vi "Baseline calculation_new.vi"(4 "Sampling rate":dbl=10000.0 format="%#_13g", 5 "Data type":T2 items=["AXON", "HEKA"], 7 "Event Detection (1D)":T1[](array[typedef])) -> (3 "Baseline info":cluster{dbl[][]}[](array[cluster]))   [LabVIEW 2017]
uses:
  Data type_new.ctl
  Event Detection cluster.ctl
  <vilib>/Analysis/baseanly.llb/Mean (DBL).vi
  <vilib>/Analysis/NI_AALBase.lvlib
  <vilib>/Analysis/NI_AALPro.lvlib
panel:
  out "Event Detection (1D) OUT":T1[](array[typedef])
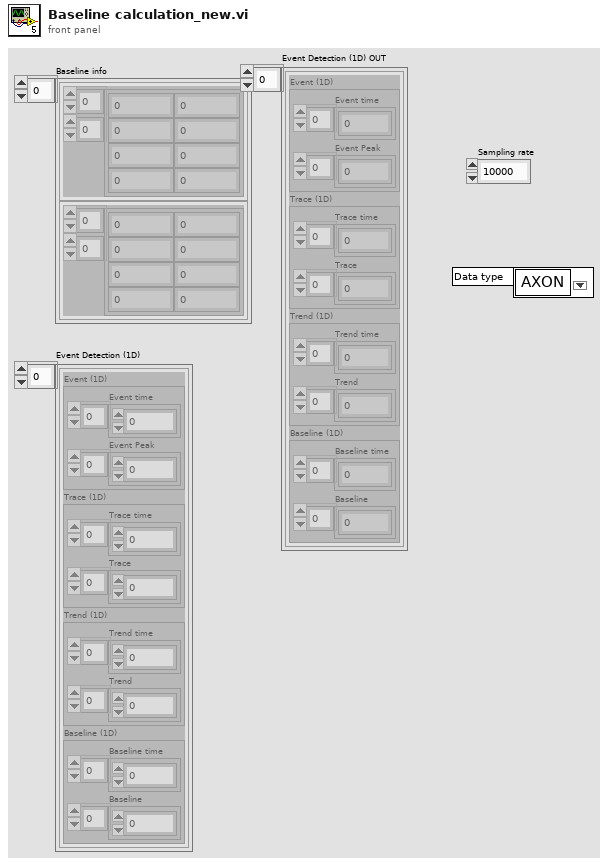
[diagram p1: front panel]
types:
  T1 = typedef "Event Detection cluster.ctl" = cluster{"Event (1D)":cluster{"Event time":dbl[], "Event Peak":dbl[]}, "Trace (1D)":cluster{"Trace time":dbl[], "Trace":dbl[]}, "Trend (1D)":cluster{"Trend time":dbl[], "Trend":dbl[]}, "Baseline (1D)":cluster{"Baseline time":dbl[], "Baseline":dbl[]}}
  T2 = typedef "Data type_new.ctl" = u16
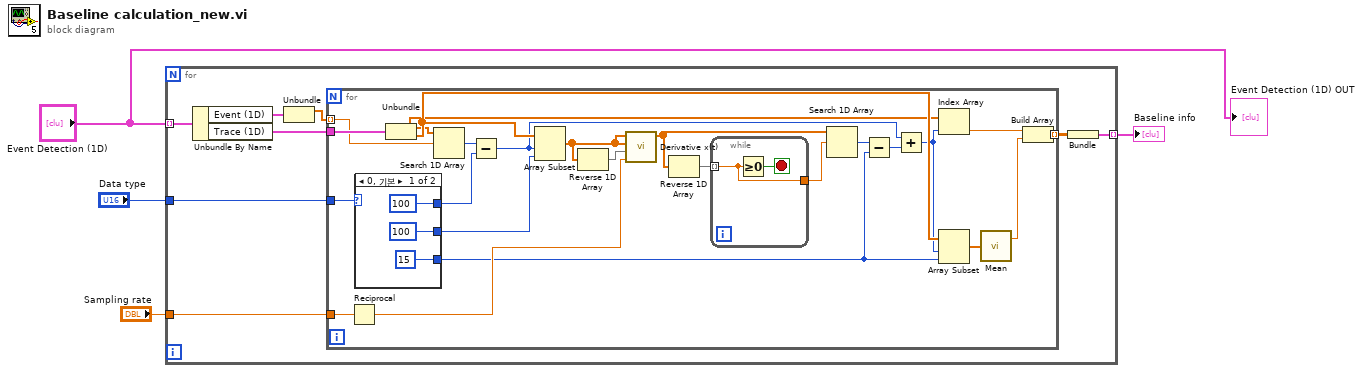
[diagram p0: block diagram]
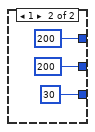
[diagram p2: hidden frame]
diagram:
  n1 = for {
    tunnel: "Data type" -> [w12]
    tunnel: [w10] -> w3 mode=indexing
    tunnel: "Event Detection (1D)" -> [w9] mode=indexing
    tunnel: "Sampling rate" -> [w5]
    n2 = Unbundle By Name(w9) -> ("Event (1D)"=w8:cluster{"Event time":dbl[], "Event Peak":dbl[]}, "Trace (1D)"=w6:cluster{"Trace time":dbl[], "Trace":dbl[]})
    n3 = Unbundle(w8) -> ("Event time"=w7:dbl[])  [unwired: 1 out]
    n4 = for {
      tunnel: w6 -> [w36]
      tunnel: w12 -> [w33]
      tunnel: [w24] -> w11 mode=indexing
      tunnel: w7 -> [w14] mode=indexing
      tunnel: w5 -> [w13]
      n5 = Reciprocal(x=w13) -> (1/x=w31:dbl)
      n6 = case shown="0, 기본" w33 {
        tunnel: [100 ("y") 200 ("y")] -> w35
        tunnel: [100 ("길이") 200 ("길이")] -> w34
        tunnel: [15 ("y") 30 ("y")] -> w15
        frame 0, Default {
        }
        frame 1 {
        }
      }
      n7 = Unbundle(w36) -> ("Trace time"=w21:dbl[], "Trace"=w28:dbl[])
      n8 = Search 1D Array(1D array=w21, element=w14) -> (index of element=w19:i32)  [unwired: 1 in]
      n9 = Subtract(x=w19, y=w35) -> (x-y=w17:i32)
      n10 = Array Subset(array=w28, index=w17, length=w34) -> (w23:dbl[])
      n11 = Reverse 1D Array(array=w23) -> (reversed array=w32:dbl[])
      n12 = call <vilib>:"Derivative x(t).vi"("dt"=w31, "Final Condition"=w32, "Initial Condition"=w23, "X"=w23) -> ("dX/dt"=w22:dbl[])  [unwired: 6 in, 1 out]
      n13 = Reverse 1D Array(array=w22) -> (reversed array=w30:dbl[])
      n14 = while {
        tunnel: w30 -> [w37] mode=indexing
        tunnel: [w37] -> w29
        stop <- w38 stop-if-true
        n15 = Greater Or Equal To 0?(x=w37) -> (x >= 0?=w38:bool)
      }
      n16 = Search 1D Array(1D array=w22, element=w29) -> (index of element=w20:i32)  [unwired: 1 in]
      n17 = Subtract(x=w20, y=w15) -> (x-y=w18:i32)
      n18 = Add(x=w17, y=w18) -> (x+y=w16:i32)
      n19 = Index Array(array=w21, index=w16) -> (element=w27:dbl)
      n20 = Array Subset(array=w28, index=w16, length=w15) -> (w26:dbl[])
      n21 = call-poly <vilib>:"Mean.vi"("X"=w26) -> ("mean"=w25:dbl)  [unwired: 1 out]
      n22 = Build Array(w27, w25) -> (w24:dbl[])
    }
    n23 = Bundle(w11) -> (w10:cluster{dbl[][]})  [unwired: 1 in]
  }
  "Baseline info" <- w3
  "Event Detection (1D) OUT" <- "Event Detection (1D)"
